vi "Acquisition + IR (Event).vi"() -> ()   [LabVIEW 2010]
uses:
  wiimotestate.ctl
  wiimoteState(IR).ctl
  C:/Users/×ñÞóôïò/Desktop/rtdsp_project14_4_11/3D_Experiment/libs/ola/WiimoteManaged(wml17)/WiimoteLib.dll
  WiimoteLib.dll
panel:
  out "IR Camera Targets":picture
  out "Cluster":cluster{"Wiimote State":T1, "IRState":T2} {"IRState"."Mode" items=["Off"=0, "Basic"=1, "Extended"=3, "Full"=5]}
  in  "stop":bool
  out "error out":errorcluster
  # "Establish a Bluetooth link with your Wiimote prior to executing this VI.\n\nRequires the Wiimote Managed Library WiimoteLib Ver 1.7\navailable from http://www.codeplex.com/WiimoteLib\nSam Shearman"
  # "Accelerometers"
  # "Buttons"
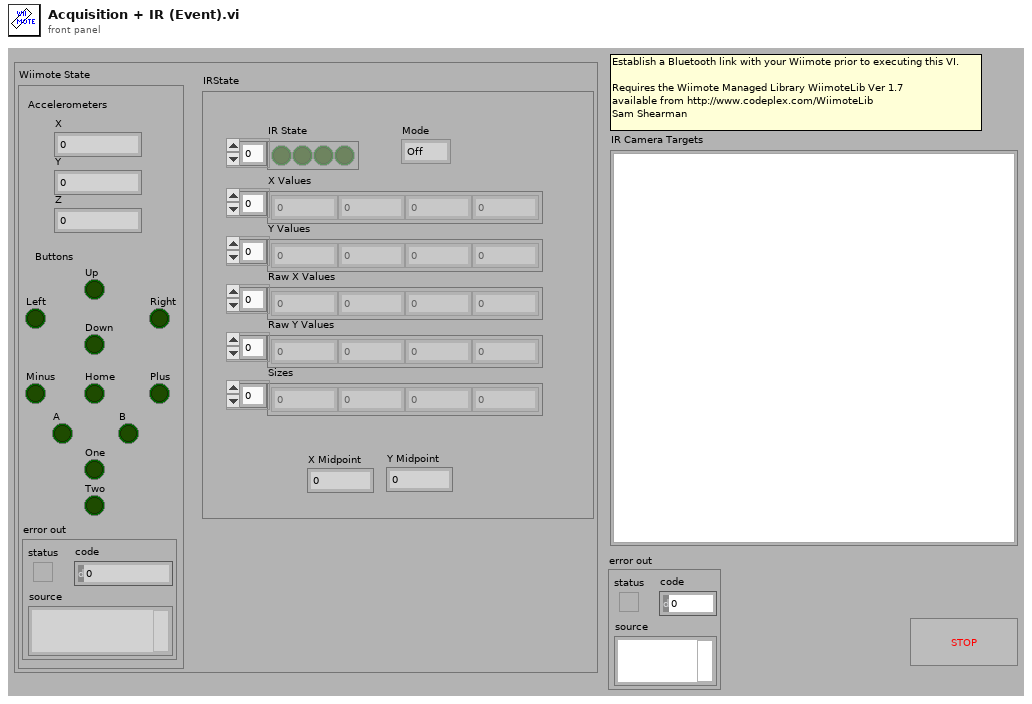
[diagram p1: front panel]
types:
  T1 = typedef "wiimotestate.ctl" = cluster{"X":sgl, "Y":sgl, "Z":sgl, "A":bool, "B":bool, "Down":bool, "Home":bool, "Left":bool, "Minus":bool, "One":bool, "Plus":bool, "Right":bool, "Two":bool, "Up":bool, "error out":errorcluster}
  T2 = typedef "wiimoteState(IR).ctl" = cluster{"Mode":u8, "IR State":bool[], "X Values":sgl[], "Y Values":sgl[], "Raw X Values":i32[], "Raw Y Values":i32[], "Sizes":i32[], "X Midpoint":sgl, "Y Midpoint":sgl}
  T3 = typedef "LVBoundsTypeDef.ctl" = cluster{"Width":u32, "Height":u32}
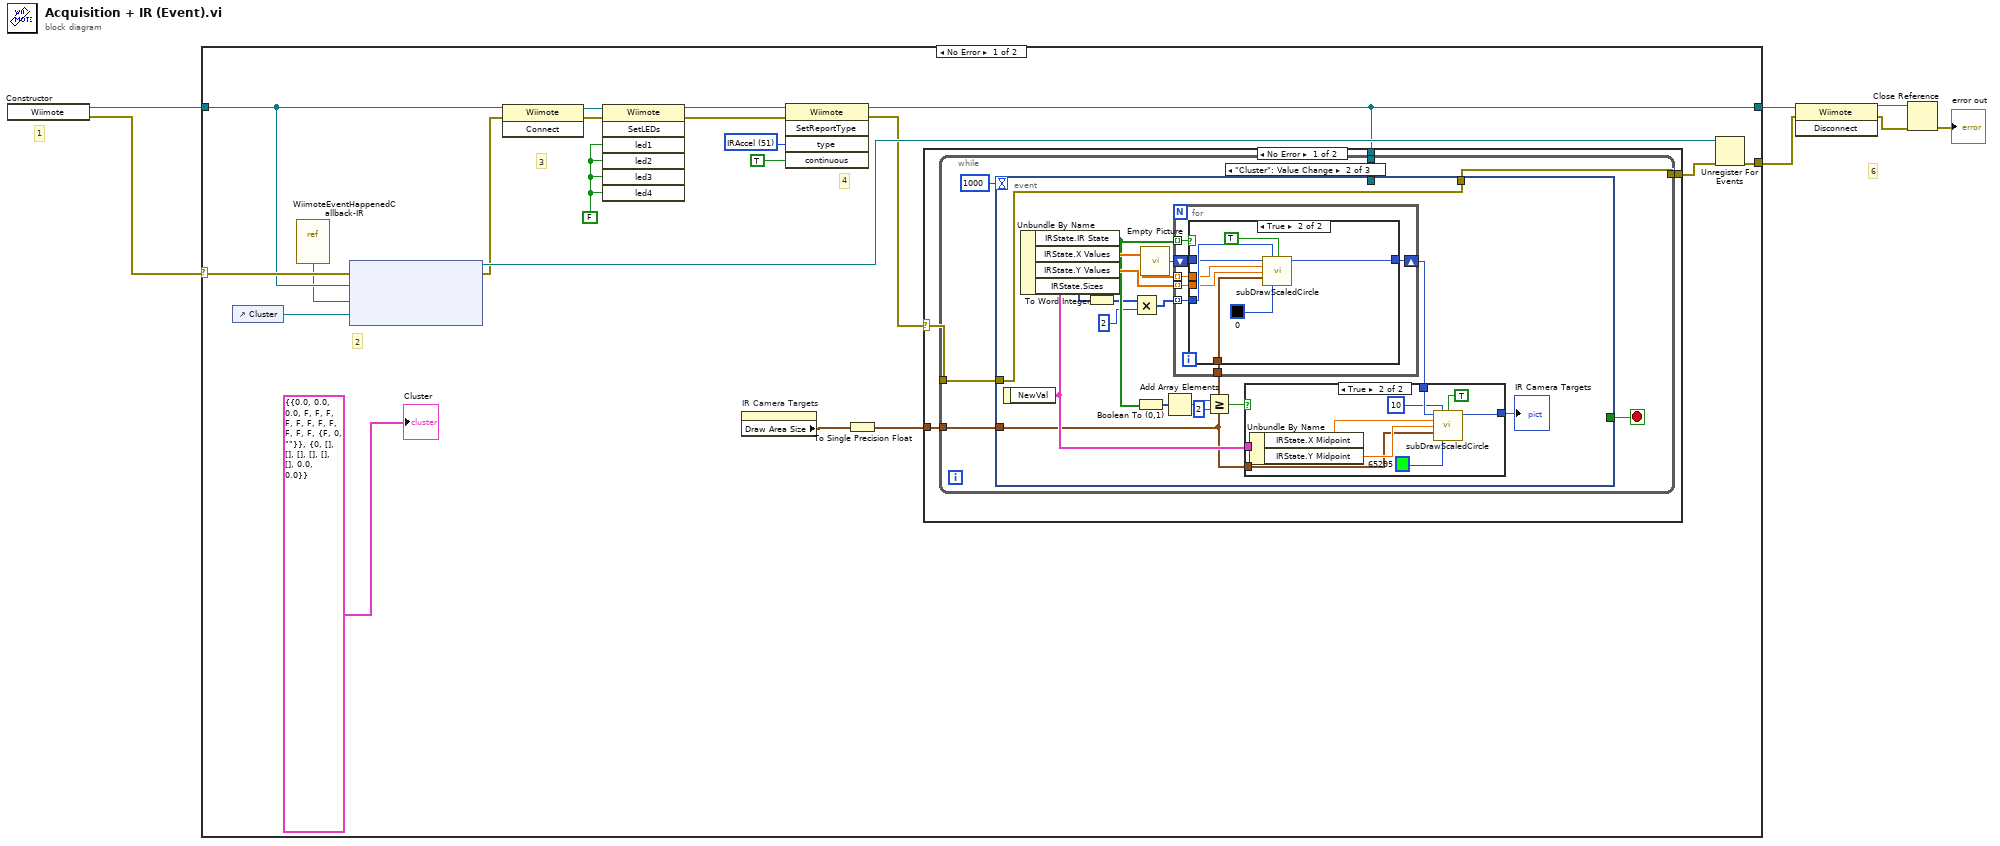
[diagram p0: block diagram]
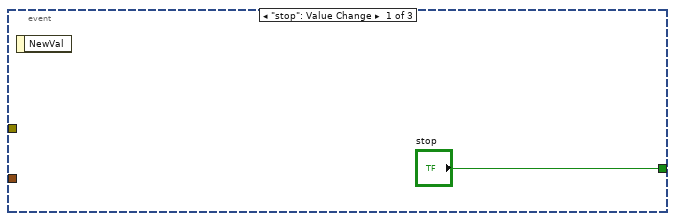
[diagram p2: hidden frame]
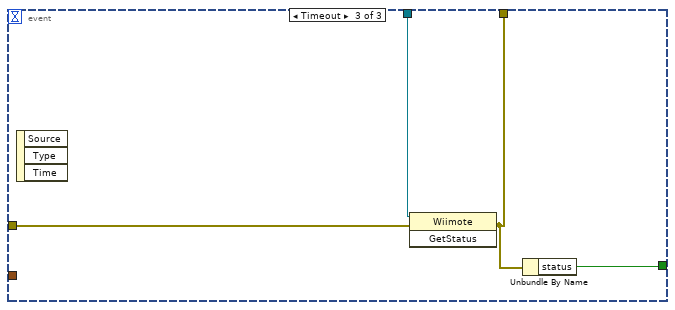
[diagram p5: hidden frame]
diagram:
  # "6"
  # "1"
  n1 = constructor class="Wiimote"() -> (reference out=w2:refnum<k24>, error out=w1:errorcluster)  [unwired: 3 in, 1 out]
  n2 = case shown="No Error" w1 {
    selector: w1 -> [w21 w88]
    tunnel: [w26 w88] -> w5
    tunnel: [w20 w87] -> w3
    tunnel: w2 -> [w10 w87]
    frame No Error {
      w23 = u8 51 items=["Status"=32, "ReadData"=33, "Buttons"=48, "ButtonsAccel"=49, "IRAccel"=51, "ButtonsExtension"=52, "ExtensionAccel"=53, "IRExtensionAccel"=55] ("type")
      w17 = FALSE ("continuous")
      # "2"
      # "4"
      # "3"
      n3 = control-ref of="Cluster"() -> (w27:refnum<vi>)
      n4 = vi-ref "WiimoteEventHappenedCallback-IR.vi"() -> ("vi reference"=w8:refnum<vi>)
      n5 = node(w21, w10, w8, w27) -> (w24:refnum<k27>, w19:errorcluster)  [unwired: 1 in]
      n6 = invoke class="Wiimote" method="Connect"(reference=w10, error in=w19) -> (reference out=w18:refnum<k24>, error out=w15:errorcluster)  [unwired: 1 in, 1 out]
      n7 = invoke class="Wiimote" method="SetLEDs"(reference=w18, error in=w15, "led1"=w17, "led2"=w17, "led3"=w17, "led4"=w17) -> (reference out=w16:refnum<k24>, error out=w14:errorcluster)  [unwired: 1 in, 5 out]
      n8 = property on="IR Camera Targets" class="Pict"() -> ("Draw Area Size"=w12:T3)  [unwired: 2 in, 2 out]
      n9 = invoke class="Wiimote" method="SetReportType"(reference=w16, error in=w14, "type"=w23, "continuous"=TRUE) -> (reference out=w20:refnum<k24>, error out=w11:errorcluster)  [unwired: 1 in, 3 out]
      n10 = To Single Precision Float(number=w12) -> (single precision float=w13:cluster{"Width":sgl, "Height":sgl})
      n11 = case shown="No Error" w11 {
        selector: w11 -> [w28 w86]
        tunnel: [w31 w86] -> w25
        tunnel: w20 -> [w30 _]
        tunnel: w13 -> [w29 _]
        frame No Error {
          n12 = while {
            tunnel: [w33] -> w31
            tunnel: w28 -> [w36]
            tunnel: w30 -> [w35]
            tunnel: w29 -> [w32]
            stop <- w37 stop-if-true
            n13 = event shown="[1] \"Cluster\": Value Change" {
              selector: _ -> [_ _ _]
              dyn-events: _ -> [_ _ _]
              timeout: 1000 -> [_ _ _]
              tunnel: ["stop" _ w83] -> w37
              tunnel: w36 -> [_ w48 w85]
              tunnel: w35 -> [_ _ w84]
              tunnel: [_ w48 w82] -> w33
              tunnel: w32 -> [_ w49 _]
              event "stop": Value Change {
                n14 = event-data() -> ()  [unwired: 2 out]
              }
              event "Cluster": Value Change {
                n15 = event-data() -> ("NewVal"=w52:cluster{"Wiimote State":T1, "IRState":T2})  [unwired: 1 out]
                n16 = Unbundle By Name(w52) -> ("IRState.IR State"=w47:bool[], "IRState.X Values"=w53:sgl[], "IRState.Y Values"=w54:sgl[], "IRState.Sizes"=w42:i32[])
                n17 = To Word Integer(number=w42) -> (16bit integer=w39:i16[])
                n18 = Multiply(x=w39, y=i16 2) -> (x*y=w41:i16[])
                n19 = Boolean To (0,1)(Boolean=w47) -> (0, 1=w46:i16[])
                n20 = call "Empty Picture"() -> ("empty picture"=w55:picture)
                n21 = Add Array Elements(numeric array=w46) -> (sum=w44:i16)
                n22 = for {
                  shift-right: [w71] -> w50
                  shift-left: w55 -> [w72]
                  tunnel: w41 -> [w70] mode=indexing
                  tunnel: w53 -> [w69] mode=indexing
                  tunnel: w54 -> [w68] mode=indexing
                  tunnel: w49 -> [w67]
                  tunnel: w47 -> [w66] mode=indexing
                  n23 = case shown="True" w66 {
                    tunnel: w72 -> [w73 w76]
                    tunnel: [w73 w81] -> w71
                    tunnel: w70 -> [_ w77]
                    tunnel: w69 -> [_ w75]
                    tunnel: w68 -> [_ w74]
                    tunnel: w67 -> [_ w80]
                    frame False {
                    }
                    frame True {
                      n24 = call "subDrawScaledCircle.vi"("picture in"=w76, "Radius"=w77, "fill?(F)"=TRUE, "X"=w75, "Y"=w74, "Display Size"=w80, "color(black)"=u32 0) -> ("picture out"=w81:picture)  [unwired: 1 in, 7 out]
                    }
                  }
                }
                n25 = Greater Or Equal?(x=w44, y=i16 2) -> (x >= y?=w45:bool)
                n26 = case shown="True" w45 {
                  tunnel: w52 -> [_ w65]
                  tunnel: [w56 w60] -> w51
                  tunnel: w50 -> [w56 w61]
                  tunnel: w49 -> [_ w58]
                  frame False {
                  }
                  frame True {
                    n27 = Unbundle By Name(w65) -> ("IRState.X Midpoint"=w64:sgl, "IRState.Y Midpoint"=w63:sgl)
                    n28 = call "subDrawScaledCircle.vi"("picture in"=w61, "Radius"=i16 10, "fill?(F)"=TRUE, "X"=w64, "Y"=w63, "Display Size"=w58, "color(black)"=u32 65295) -> ("picture out"=w60:picture)  [unwired: 1 in, 7 out]
                  }
                }
                "IR Camera Targets" <- w51
              }
              event Timeout {
                n29 = event-data() -> ()  [unwired: 4 out]
                n30 = invoke class="Wiimote" method="GetStatus"(reference=w84, error in=w85) -> (error out=w82:errorcluster)  [unwired: 1 in, 2 out]
                n31 = Unbundle By Name(w82) -> ("status"=w83:bool)
              }
            }
          }
        }
        frame Error {
        }
      }
      n32 = Unregister For Events(event registration refnum=w24, error in=w25) -> (error out=w26:errorcluster)
      "Cluster" <- cluster{"Wiimote State":T1, "IRState":T2} {"Wiimote State"={"X"=0.0, "Y"=0.0, "Z"=0.0, "A"=FALSE, "B"=FALSE, "Down"=FALSE, "Home"=FALSE, "Left"=FALSE, "Minus"=FALSE, "One"=FALSE, "Plus"=FALSE, "Right"=FALSE, "Two"=FALSE, "Up"=FALSE, "error out"={"status"=FALSE, "code"=0, "source"=""}}, "IRState"={"Mode"=0, "IR State"=[], "X Values"=[], "Y Values"=[], "Raw X Values"=[], "Raw Y Values"=[], "Sizes"=[], "X Midpoint"=0.0, "Y Midpoint"=0.0}} ("Cluster")
    }
    frame Error {
    }
  }
  n33 = invoke class="Wiimote" method="Disconnect"(reference=w3, error in=w5) -> (reference out=w7:refnum<k24>, error out=w4:errorcluster)  [unwired: 1 in, 1 out]
  n34 = Close Reference(reference=w7, error in (no error)=w4) -> (error out=→"error out":errorcluster)
